vi "Manager QuerySystemStatus.vi"(6 "contextId":T1, 8 "error in":errorcluster, 9 "timeout (ms)":i32=-1, 10 "Request Data":T6, 11 "gRPC ID":T1) -> (0 "error out":errorcluster, 2 "Response Data":T2, 3 "gRPC ID out":T1)   [LabVIEW 2021, in "CIF_Manager_client.lvlib"]
uses:
  CIF_Manager_client.lvlib
  <vilib>/gRPC/LabVIEW gRPC Library/Shared/grpcId.ctl
  RPC Messages/cif_manager_PluginStatus.ctl
  RPC Messages/cif_manager_PluginName.ctl
  RPC Messages/cif_plugincore_StatusData.ctl
  RPC Messages/cif_plugincore_StatusData_PluginState.ctl
  RPC Messages/cif_plugincore_TimingStatistics.ctl
  RPC Messages/cif_common_TimingStats.ctl
  RPC Messages/cif_plugincore_FifoStatistics.ctl
  RPC Messages/cif_plugincore_Error.ctl
  RPC Messages/cif_plugincore_MonitorDoubles.ctl
  RPC Messages/cif_plugincore_MonitorU64.ctl
  RPC Messages/cif_plugincore_MonitorI64.ctl
  RPC Messages/cif_channelcore_Channels.ctl
  RPC Messages/cif_channelcore_Channel.ctl
  RPC Messages/cif_channelcore_ChannelDirection.ctl
  RPC Messages/cif_channelcore_ChannelPattern.ctl
  RPC Messages/cif_manager_SystemStatus.ctl
  RPC Messages/cif_manager_ClockConversionArray.ctl
  RPC Messages/cif_manager_ClockConversion.ctl
  RPC Messages/cif_manager_TimePair.ctl
  RPC Messages/cif_manager_SystemStatus_Flat.ctl
  RPC Messages/cif_manager_ClockConversionArray_Flat.ctl
  RPC Messages/cif_manager_ClockConversion_Flat.ctl
  RPC Messages/cif_manager_TimePair_Flat.ctl
  14035477-4c25-4107-8ed5-d0c4ef420ce5.vi
  RPC Messages/RichToFlatcif_manager_PluginName.vi
  RPC Messages/RichToFlatcif_plugincore_StatusData.vi
  RPC Messages/RichToFlatcif_channelcore_Channels.vi
  <vilib>/gRPC/LabVIEW gRPC Library/Shared/TranslateGrpcError.vi
  <vilib>/gRPC/LabVIEW gRPC Library/Shared/Wait On Occurrence.vi
  RPC Messages/FlatToRichcif_manager_ClockConversionArray.vi
  RPC Messages/RichToFlatcif_plugincore_TimingStatistics.vi
  RPC Messages/RichToFlatcif_plugincore_FifoStatistics.vi
  RPC Messages/RichToFlatcif_plugincore_Error.vi
  RPC Messages/RichToFlatcif_plugincore_MonitorDoubles.vi
  RPC Messages/RichToFlatcif_plugincore_MonitorU64.vi
  RPC Messages/RichToFlatcif_plugincore_MonitorI64.vi
  RPC Messages/RichToFlatcif_channelcore_Channel.vi
  <vilib>/gRPC/LabVIEW gRPC Library/Shared/Is Feature Enabled.vi
  RPC Messages/FlatToRichcif_manager_ClockConversion.vi
  RPC Messages/RichToFlatcif_common_TimingStats.vi
  RPC Messages/FlatToRichcif_manager_TimePair.vi
  <vilib>/gRPC/LabVIEW gRPC Library/Server API/Server/Get Server DLL Path.vi
  <vilib>/Utility/error.llb/Error Cluster From Error Code.vi
  <vilib>/gRPC/LabVIEW gRPC Library/grpc-lvsupport-release.lvlib
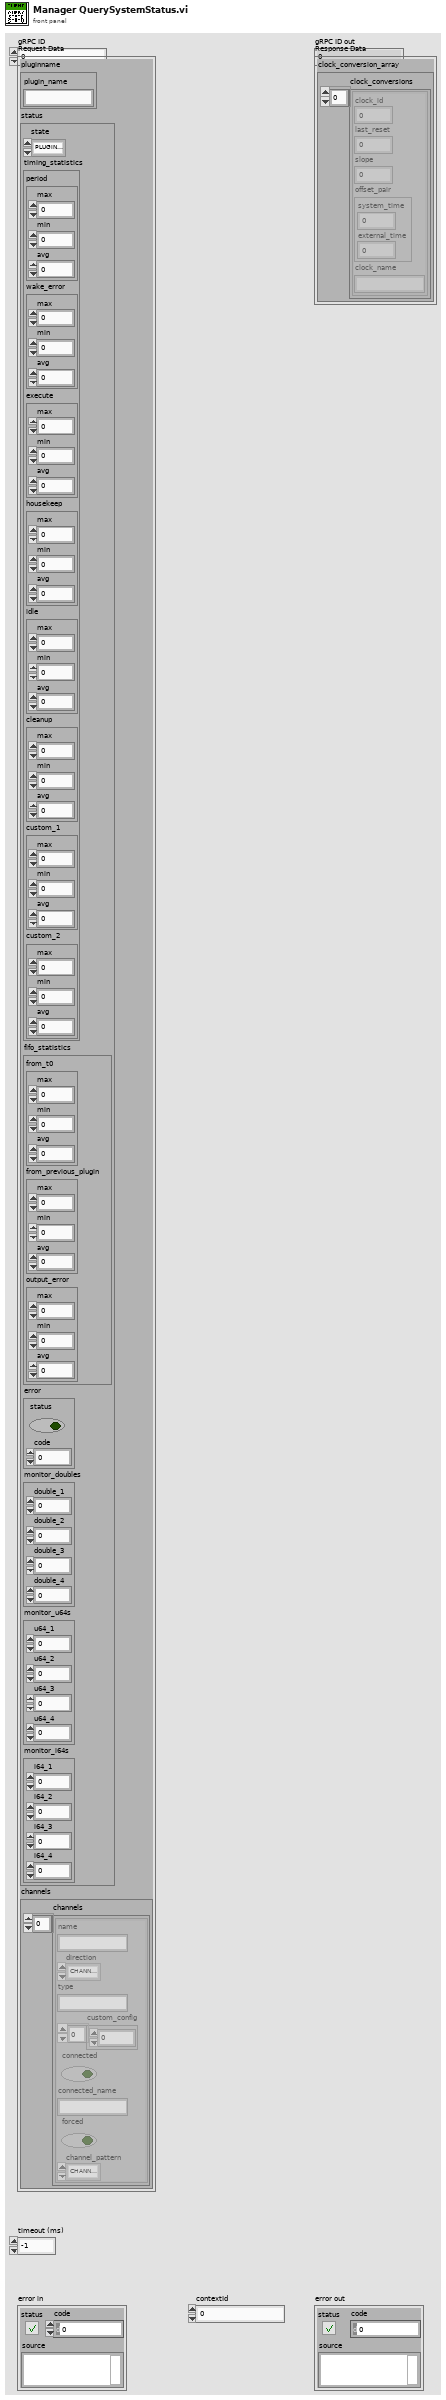
[diagram p1: front panel]
types:
  T1 = typedef "grpc-lvsupport-release.lvlib/grpcId.ctl" = u64
  T2 = typedef "CIF_Manager_client.lvlib/cif_manager_SystemStatus.ctl" = cluster{"clock_conversion_array":T3}
  T3 = typedef "CIF_Manager_client.lvlib/cif_manager_ClockConversionArray.ctl" = cluster{"clock_conversions":T4[]}
  T4 = typedef "CIF_Manager_client.lvlib/cif_manager_ClockConversion.ctl" = cluster{"clock_id":u32, "last_reset":i64, "slope":dbl, "offset_pair":T5, "clock_name":string}
  T5 = typedef "CIF_Manager_client.lvlib/cif_manager_TimePair.ctl" = cluster{"system_time":i64, "external_time":i64}
  T6 = typedef "CIF_Manager_client.lvlib/cif_manager_PluginStatus.ctl" = cluster{"pluginname":T7, "status":T8, "channels":T17}
  T7 = typedef "CIF_Manager_client.lvlib/cif_manager_PluginName.ctl" = cluster{"plugin_name":string}
  T8 = typedef "CIF_Manager_client.lvlib/cif_plugincore_StatusData.ctl" = cluster{"state":T9, "timing_statistics":T10, "fifo_statistics":T12, "error":T13, "monitor_doubles":T14, "monitor_u64s":T15, "monitor_i64s":T16}
  T9 = typedef "CIF_Manager_client.lvlib/cif_plugincore_StatusData_PluginState.ctl" = enum32{"PLUGINSTATE_UNKNOWN", "PLUGINSTATE_CREATING", "PLUGINSTATE_LISTENING", "PLUGINSTATE_RUNNING", "PLUGINSTATE_CLEANINGUP", "PLUGINSTATE_DESTROYING"}
  T10 = typedef "CIF_Manager_client.lvlib/cif_plugincore_TimingStatistics.ctl" = cluster{"period":T11, "wake_error":T11, "execute":T11, "housekeep":T11, "idle":T11, "cleanup":T11, "custom_1":T11, "custom_2":T11}
  T11 = typedef "CIF_Manager_client.lvlib/cif_common_TimingStats.ctl" = cluster{"max":i64, "min":i64, "avg":dbl}
  T12 = typedef "CIF_Manager_client.lvlib/cif_plugincore_FifoStatistics.ctl" = cluster{"from_t0":T11, "from_previous_plugin":T11, "output_error":T11}
  T13 = typedef "CIF_Manager_client.lvlib/cif_plugincore_Error.ctl" = cluster{"status":bool, "code":i32}
  T14 = typedef "CIF_Manager_client.lvlib/cif_plugincore_MonitorDoubles.ctl" = cluster{"double_1":dbl, "double_2":dbl, "double_3":dbl, "double_4":dbl}
  T15 = typedef "CIF_Manager_client.lvlib/cif_plugincore_MonitorU64.ctl" = cluster{"u64_1":u64, "u64_2":u64, "u64_3":u64, "u64_4":u64}
  T16 = typedef "CIF_Manager_client.lvlib/cif_plugincore_MonitorI64.ctl" = cluster{"i64_1":i64, "i64_2":i64, "i64_3":i64, "i64_4":i64}
  T17 = typedef "CIF_Manager_client.lvlib/cif_channelcore_Channels.ctl" = cluster{"channels":T18[]}
  T18 = typedef "CIF_Manager_client.lvlib/cif_channelcore_Channel.ctl" = cluster{"name":string, "direction":T19, "type":string, "custom_config":u8[], "connected":bool, "connected_name":string, "forced":bool, "channel_pattern":T20}
  T19 = typedef "CIF_Manager_client.lvlib/cif_channelcore_ChannelDirection.ctl" = enum32{"CHANNELDIRECTION_UNKNOWN", "CHANNELDIRECTION_PUBLISHER", "CHANNELDIRECTION_SUBSCRIBER"}
  T20 = typedef "CIF_Manager_client.lvlib/cif_channelcore_ChannelPattern.ctl" = enum32{"CHANNELPATTERN_UNKNOWN", "CHANNELPATTERN_TAG", "CHANNELPATTERN_FIFO", "CHANNELPATTERN_MULTIFIFO", "CHANNELPATTERN_BACKPRESSUREFIFO"}
  T21 = typedef "CIF_Manager_client.lvlib/cif_manager_SystemStatus_Flat.ctl" = cluster{"clock_conversion_array":T22}
  T22 = typedef "CIF_Manager_client.lvlib/cif_manager_ClockConversionArray_Flat.ctl" = cluster{"clock_conversions":T23[]}
  T23 = typedef "CIF_Manager_client.lvlib/cif_manager_ClockConversion_Flat.ctl" = cluster{"clock_id":u32, "last_reset":i64, "slope":dbl, "offset_pair":T24, "clock_name":string}
  T24 = typedef "CIF_Manager_client.lvlib/cif_manager_TimePair_Flat.ctl" = cluster{"system_time":i64, "external_time":i64}
  T25 = typedef "CIF_Manager_client.lvlib/cif_manager_PluginStatus_Flat.ctl" = cluster{"pluginname":T26, "status":T27, "channels":T35}
  T26 = typedef "CIF_Manager_client.lvlib/cif_manager_PluginName_Flat.ctl" = cluster{"plugin_name":string}
  T27 = typedef "CIF_Manager_client.lvlib/cif_plugincore_StatusData_Flat.ctl" = cluster{"state":T9, "timing_statistics":T28, "fifo_statistics":T30, "error":T31, "monitor_doubles":T32, "monitor_u64s":T33, "monitor_i64s":T34}
  T28 = typedef "CIF_Manager_client.lvlib/cif_plugincore_TimingStatistics_Flat.ctl" = cluster{"period":T29, "wake_error":T29, "execute":T29, "housekeep":T29, "idle":T29, "cleanup":T29, "custom_1":T29, "custom_2":T29}
  T29 = typedef "CIF_Manager_client.lvlib/cif_common_TimingStats_Flat.ctl" = cluster{"max":i64, "min":i64, "avg":dbl}
  T30 = typedef "CIF_Manager_client.lvlib/cif_plugincore_FifoStatistics_Flat.ctl" = cluster{"from_t0":T29, "from_previous_plugin":T29, "output_error":T29}
  T31 = typedef "CIF_Manager_client.lvlib/cif_plugincore_Error_Flat.ctl" = cluster{"status":bool, "code":i32}
  T32 = typedef "CIF_Manager_client.lvlib/cif_plugincore_MonitorDoubles_Flat.ctl" = cluster{"double_1":dbl, "double_2":dbl, "double_3":dbl, "double_4":dbl}
  T33 = typedef "CIF_Manager_client.lvlib/cif_plugincore_MonitorU64_Flat.ctl" = cluster{"u64_1":u64, "u64_2":u64, "u64_3":u64, "u64_4":u64}
  T34 = typedef "CIF_Manager_client.lvlib/cif_plugincore_MonitorI64_Flat.ctl" = cluster{"i64_1":i64, "i64_2":i64, "i64_3":i64, "i64_4":i64}
  T35 = typedef "CIF_Manager_client.lvlib/cif_channelcore_Channels_Flat.ctl" = cluster{"channels":T36[]}
  T36 = typedef "CIF_Manager_client.lvlib/cif_channelcore_Channel_Flat.ctl" = cluster{"name":string, "direction":T19, "type":string, "custom_config":u8[], "connected":bool, "connected_name":string, "forced":bool, "channel_pattern":T20}
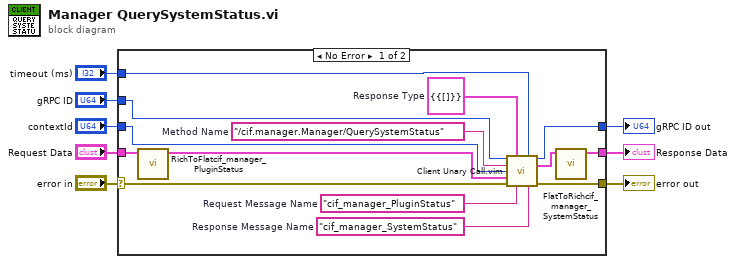
[diagram p0: block diagram]
diagram:
  n1 = case shown="No Error" "error in" {
    selector: "error in" -> [w18 w23]
    tunnel: [w17 w23] -> w7
    tunnel: "gRPC ID" -> [w16 w24]
    tunnel: [w15 w24] -> w5
    tunnel: "Request Data" -> [w12 _]
    tunnel: [w9 _] -> w3
    tunnel: "timeout (ms)" -> [w14 _]
    tunnel: "contextId" -> [w13 _]
    frame No Error {
      w19 = "cif_manager_SystemStatus"  # Response Message Name
      w20 = "cif_manager_PluginStatus"  # Request Message Name
      w21 = T21 {"clock_conversion_array"={"clock_conversions"=[]}}  # Response Type
      w22 = "/cif.manager.Manager/QuerySystemStatus"  # Method Name
      n2 = call "RichToFlatcif_manager_PluginStatus.vi"("InputCluster"=w12) -> ("OutputCluster"=w11:T25)  [unwired: 10 in]
      n3 = call "Client Unary Call.vim"("ClientID in"=w16, "Response Type"=w21, "timeout (ms)"=w14, "Method Name"=w22, "contextId"=w13, "Request Data"=w11, "error in"=w18, "Request Message Name"=w20, "Response Message Name"=w19) -> ("ClientID out"=w15:u64, "Response Data"=w10:T21, "error out"=w17:errorcluster)  [unwired: 4 in]
      n4 = call "FlatToRichcif_manager_SystemStatus.vi"("InputCluster"=w10) -> ("OutputCluster"=w9:T2)  [unwired: 10 in]
    }
    frame Error {
    }
  }
  "error out" <- w7
  "gRPC ID out" <- w5
  "Response Data" <- w3
